vi "Remove Step From Tree.vi"(10 "Step Index":i32, 11 "TreeControl in":refnum<vi>) -> (3 "TreeControl out":refnum<vi>)   [LabVIEW 2020, in "Output Sequencer.lvlib" / "Settings UI.lvclass"]
uses:
  Settings UI.lvclass
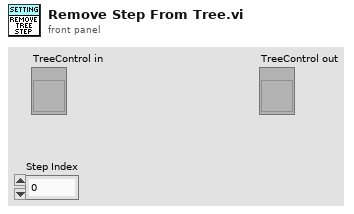
[diagram p1: front panel]
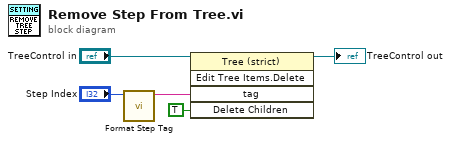
[diagram p0: block diagram]
diagram:
  n1 = call "Format Step Tag.vi"("Step Number"="Step Index") -> ("Tag"=w1:string)  [unwired: 10 in]
  n2 = invoke class="Tree (strict)" method="Edit Tree Items.Delete"(reference="TreeControl in", "tag"=w1, "Delete Children"=TRUE ("Delete Children?")) -> (reference out=→"TreeControl out":refnum<vi>)  [unwired: 2 in, 4 out]
